vi "PythonToIMAQ_Image.vi"(8 "error in (no error)":errorcluster, 10 "Python Image":u8[][][](array[numeric]), 11 "IMAQ Image in":T1) -> (0 "error out":errorcluster, 3 "IMAQ Image out":T1)   [LabVIEW 2017, in "ImageFacialDetection.lvclass"]
doc: "converts a python 3D array image into a LabVIEW 2D picture"
uses:
  ImageFacialDetection.lvclass
  <vilib>/vision/Image Controls.llb/IMAQ Image.ctl
  <vilib>/picture/picture.llb/imagedata.ctl
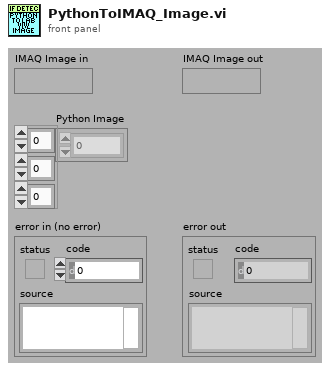
[diagram p1: front panel]
types:
  T1 = typedef "IMAQ Image.ctl" = refnum<image>
  T2 = typedef "imagedata.ctl" = cluster{"image type":i32, "image depth":i32, "image":u8[], "mask":u8[], "colors":u32[], "Rectangle":cluster{"left":i16, "top":i16, "right":i16, "bottom":i16}}
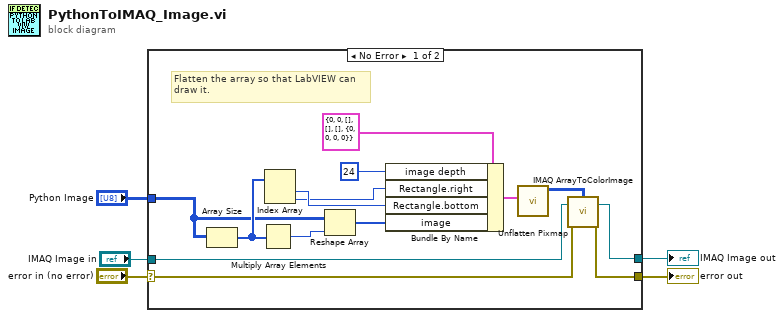
[diagram p0: block diagram]
diagram:
  n1 = case shown="No Error" "error in (no error)" {
    selector: "error in (no error)" -> [w7 w20]
    tunnel: [w6 w20] -> w4
    tunnel: "Python Image" -> [w12 _]
    tunnel: [w8 _] -> w2
    tunnel: "IMAQ Image in" -> [w9 _]
    frame No Error {
      # "Flatten the array so that LabVIEW can\ndraw it."
      n2 = Array Size(array=w12) -> (size(s)=w14:i32[])
      n3 = Multiply Array Elements(1:w14) -> (0:w13:i32)
      n4 = Index Array(array=w14) -> (element #1=w17:i32, element #2=w16:i32)  [unwired: 2 in]
      n5 = Reshape Array(w12, w13) -> (w15:u8[])
      n6 = Bundle By Name(cluster=T2 {"image type"=0, "image depth"=0, "image"=[], "mask"=[], "colors"=[], "Rectangle"={"left"=0, "top"=0, "right"=0, "bottom"=0}} ("image data"), "image depth"=24, "Rectangle.right"=w16, "Rectangle.bottom"=w17, "image"=w15) -> (w11:T2)
      n7 = call <vilib>:"Unflatten Pixmap.vi"("image data"=w11) -> ("24-bit pixmap"=w10:u32[][])  [unwired: 4 in, 6 out]
      n8 = call "IMAQ ArrayToColorImage"("Image Pixels (U32)"=w10, "Image"=w9, "error in (no error)"=w7) -> ("Image Out"=w8:T1, "error out"=w6:errorcluster)  [unwired: 2 in]
    }
    frame Error {
    }
  }
  "error out" <- w4
  "IMAQ Image out" <- w2
